vi "MIPI_RFEE_Write and Read Utility.vi"() -> ()   [LabVIEW 2013]
doc: "This VI demonstaits how to write to and read back data from a MIPI device. To run this VI:\n1) Change Resource name to the name of your HSDIO card\n2) The MIPI clock will run at <Sample Clock Rate>/<Oversample Factor>. This is 26 MHz (full rate). If your device should be run at a slower rate, decrease the sample clock rate and (or) increase the oversample rate.\n3. At 104MHz, the RTD value should be ~5 for a 1.5 meter cable. If you are running at a different clock rate or using a different length cable, adjust the RTD Compensation value so the MIPI data is stable at the falling edge of the clock. If you need futher timing adjustment, consider setting the data position to \"Delay from Sample Clock Rising Edge\" and configuring this delay."
uses:
  MIPI_RFFE/Ctrls/Configuration.ctl
  MIPI_RFFE/Ctrls/ClockDataChannels.ctl
  <instrlib>/niHSDIO/niHSDIO.llb/niHSDIO_ctl Sample Clock Source Values (ComboBox).ctl
  <instrlib>/niHSDIO/niHSDIO.llb/niHSDIO_ctl Voltage Logic Family Values (Ring).ctl
  MIPI_RFFE/Ctrls/RegReadWrite.ctl
  <instrlib>/niHSDIO/niHSDIO.llb/niHSDIO_ctl Data Position Values (Ring).ctl
  MIPI_RFFE/Ctrls/ExtendedRegReadWrite.ctl
  <instrlib>/niHSDIO/niHSDIO.llb/niHSDIO Configure Data Voltage Logic Family.vi
  <instrlib>/niHSDIO/niHSDIO.llb/niHSDIO Configure Digital Edge Start Trigger.vi
  <instrlib>/niHSDIO/niHSDIO.llb/niHSDIO Configure Initial State (String).vi
  <instrlib>/niHSDIO/niHSDIO.llb/niHSDIO Configure Idle State (String).vi
  <instrlib>/niHSDIO/niHSDIO.llb/niHSDIO Write Named Waveform (WDT).vi
  <instrlib>/niHSDIO/niHSDIO.llb/niHSDIO Fetch Waveform (WDT).vi
  <vilib>/Waveform/DWDTOps.llb/DWDT Append Digital Signals.vi
panel:
  in  "Filename":string
  in  "Save .HWS?":bool
  in  "file path":path=path "C:/Users/er080167/Documents/AD4125E/Waveforms/Converted Waveforms"
  in  "channel list (all:\"\")":string="4,6"
  in  "delay (0.000)":dbl format="%.3f"
  out "Parity Error":bool
  out "MIPI Data Read from DUT":cluster{"Read Data":u8[]}[](array[cluster])=[{"Read Data"=[128]}] {"Read Data" format="%.0x"}
  in  "Register Read/Write":T1={"Slave Address"=6, "Register"=28, "Data"=128} {"Data" format="%.0x"; "Register" format="%.0x"; "Slave Address" max=15 format="%.0x"}
  in  "RTD Compensation Value":i32=1 min=0 max=29
  out "Digital Waveform Graph":digitalwaveform(graph)={"t0"=timestamp(3585852840.1106524 s since 1904-01-01), "dt"=5e-07, "Y"={"transitions"=[], "data"=[[1, 0, 1, 0], [1, 0, 1, 0], [1, 0, 1, 0], [1, 0, 1, 0], [1, 0, 1, 0], [1, 0, 1, 0], [1, 0, 1, 0], [1, 0, 1, 0], [0, 0, 0, 0], [0, 0, 0, 0], [0, 0, 0, 0], [0, 0, 0, 0], [0, 0, 0, 0], [0, 0, 0, 0], [0, 0, 0, 0], [0, 0, 0, 0], [0, 1, 0, 1], [0, 1, 0, 1], [0, 1, 0, 1], [0, 1, 0, 1], [0, 0, 0, 0], [0, 0, 0, 0], [0, 0, 0, 0], [0, 0, 0, 0], [1, 1, 1, 1], [1, 1, 1, 1], [1, 1, 1, 1], [1, 1, 1, 1], [1, 0, 1, 0], [1, 0, 1, 0], [1, 0, 1, 0], [1, 0, 1, 0], [1, 1, 1, 1], [1, 1, 1, 1], [1, 1, 1, 1], [1, 1, 1, 1], [1, 0, 1, 0], [1, 0, 1, 0], [1, 0, 1, 0], [1, 0, 1, 0], [0, 1, 0, 1], [0, 1, 0, 1], [0, 1, 0, 1], [0, 1, 0, 1], [0, 0, 0, 0], [0, 0, 0, 0], [0, 0, 0, 0], [0, 0, 0, 0], [0, 1, 0, 1], [0, 1, 0, 1], [0, 1, 0, 1], [0, 1, 0, 1], [0, 0, 0, 0], [0, 0, 0, 0], [0, 0, 0, 0], [0, 0, 0, 0], [1, 1, 1, 1], [1, 1, 1, 1], [1, 1, 1, 1], [1, 1, 1, 1], [1, 0, 1, 0], [1, 0, 1, 0], [1, 0, 1, 0], [1, 0, 1, 0], [0, 1, 0, 1], [0, 1, 0, 1], [0, 1, 0, 1], [0, 1, 0, 1], [0, 0, 0, 0], [0, 0, 0, 0], [0, 0, 0, 0], [0, 0, 0, 0], [1, 1, 1, 1], [1, 1, 1, 1], [1, 1, 1, 1], [1, 1, 1, 1], [1, 0, 1, 0], [1, 0, 1, 0], [1, 0, 1, 0], [1, 0, 1, 0], [1, 1, 1, 1], [1, 1, 1, 1], [1, 1, 1, 1], [1, 1, 1, 1], [1, 0, 1, 0], [1, 0, 1, 0], [1, 0, 1, 0], [1, 0, 1, 0], [1, 1, 1, 1], [1, 1, 1, 1], [1, 1, 1, 1], [1, 1, 1, 1], [1, 0, 1, 0], [1, 0, 1, 0], [1, 0, 1, 0], [1, 0, 1, 0], [0, 1, 0, 1], [0, 1, 0, 1], [0, 1, 0, 1], [0, 1, 0, 1], [0, 0, 0, 0], [0, 0, 0, 0], [0, 0, 0, 0], [0, 0, 0, 0], [0, 1, 0, 1], [0, 1, 0, 1], [0, 1, 0, 1], [0, 1, 0, 1], [0, 0, 0, 0], [0, 0, 0, 0], [0, 0, 0, 0], [0, 0, 0, 0], [1, 1, 1, 1], [1, 1, 1, 1], [1, 1, 1, 1], [1, 1, 1, 1], [1, 0, 1, 0], [1, 0, 1, 0], [1, 0, 1, 0], [1, 0, 1, 0], [1, 1, 1, 1], [1, 1, 1, 1], [1, 1, 1, 1], [1, 1, 1, 1], [1, 0, 1, 0], [1, 0, 1, 0], [1, 0, 1, 0], [1, 0, 1, 0], [0, 1, 0, 1], [0, 1, 0, 1], [0, 1, 0, 1], [0, 1, 0, 1], [0, 0, 0, 0], [0, 0, 0, 0], [0, 0, 0, 0], [0, 0, 0, 0], [0, 1, 0, 1], [0, 1, 0, 1], [0, 1, 0, 1], [0, 1, 0, 1], [0, 0, 0, 0], [0, 0, 0, 0], [0, 0, 0, 0], [0, 0, 0, 0], [0, 1, 0, 1], [0, 1, 0, 1], [0, 1, 0, 1], [0, 1, 0, 1], [0, 0, 0, 0], [0, 0, 0, 0], [0, 0, 0, 0], [0, 0, 0, 0], [0, 1, 0, 1], [0, 1, 0, 1], [0, 1, 0, 1], [0, 1, 0, 1], [0, 0, 0, 0], [0, 0, 0, 0], [0, 0, 0, 0], [0, 0, 0, 0], [0, 1, 0, 1], [0, 1, 0, 1], [0, 1, 0, 1], [0, 1, 0, 1], [0, 0, 0, 0], [0, 0, 0, 0], [0, 0, 0, 0], [0, 0, 0, 0], [0, 1, 0, 1], [0, 1, 0, 1], [0, 1, 0, 1], [0, 1, 0, 1], [0, 0, 0, 0], [0, 0, 0, 0], [0, 0, 0, 0], [0, 0, 0, 0], [0, 1, 0, 1], [0, 1, 0, 1], [0, 1, 0, 1], [0, 1, 0, 1], [0, 0, 0, 0], [0, 0, 0, 0], [0, 0, 0, 0], [0, 0, 0, 0], [0, 1, 0, 1], [0, 1, 0, 1], [0, 1, 0, 1], [0, 1, 0, 1], [0, 0, 0, 0], [0, 0, 0, 0], [0, 0, 0, 0], [0, 0, 0, 0], [0, 1, 0, 1], [0, 1, 0, 1], [0, 1, 0, 1], [0, 1, 0, 1], [0, 0, 0, 0], [0, 0, 0, 0], [0, 0, 0, 0], [0, 0, 0, 0], [1, 0, 1, 0], [1, 0, 1, 0], [1, 0, 1, 0], [1, 0, 1, 0], [1, 0, 1, 0], [1, 0, 1, 0], [1, 0, 1, 0], [1, 0, 1, 0], [0, 0, 0, 0], [0, 0, 0, 0], [0, 0, 0, 0], [0, 0, 0, 0], [0, 0, 0, 0], [0, 0, 0, 0], [0, 0, 0, 0], [0, 0, 0, 0], [0, 1, 0, 1], [0, 1, 0, 1], [0, 1, 0, 1], [0, 1, 0, 1], [0, 0, 0, 0], [0, 0, 0, 0], [0, 0, 0, 0], [0, 0, 0, 0], [1, 1, 1, 1], [1, 1, 1, 1], [1, 1, 1, 1], [1, 1, 1, 1], [1, 0, 1, 0], [1, 0, 1, 0], [1, 0, 1, 0], [1, 0, 1, 0], [1, 1, 1, 1], [1, 1, 1, 1], [1, 1, 1, 1], [1, 1, 1, 1], [1, 0, 1, 0], [1, 0, 1, 0], [1, 0, 1, 0], [1, 0, 1, 0], [0, 1, 0, 1], [0, 1, 0, 1], [0, 1, 0, 1], [0, 1, 0, 1], [0, 0, 0, 0], [0, 0, 0, 0], [0, 0, 0, 0], [0, 0, 0, 0], [0, 1, 0, 1], [0, 1, 0, 1], [0, 1, 0, 1], [0, 1, 0, 1], [0, 0, 0, 0], [0, 0, 0, 0], [0, 0, 0, 0], [0, 0, 0, 0], [1, 1, 1, 1], [1, 1, 1, 1], [1, 1, 1, 1], [1, 1, 1, 1], [1, 0, 1, 0], [1, 0, 1, 0], [1, 0, 1, 0], [1, 0, 1, 0], [1, 1, 1, 1], [1, 1, 1, 1], [1, 1, 1, 1], [1, 1, 1, 1], [1, 0, 1, 0], [1, 0, 1, 0], [1, 0, 1, 0], [1, 0, 1, 0], [1, 1, 1, 1], [1, 1, 1, 1], [1, 1, 1, 1], [1, 1, 1, 1], [1, 0, 1, 0], [1, 0, 1, 0], [1, 0, 1, 0], [1, 0, 1, 0], [1, 1, 1, 1], [1, 1, 1, 1], [1, 1, 1, 1], [1, 1, 1, 1], [1, 0, 1, 0], [1, 0, 1, 0], [1, 0, 1, 0], [1, 0, 1, 0], [1, 1, 1, 1], [1, 1, 1, 1], [1, 1, 1, 1], [1, 1, 1, 1], [1, 0, 1, 0], [1, 0, 1, 0], [1, 0, 1, 0], [1, 0, 1, 0], [0, 1, 0, 1], [0, 1, 0, 1], [0, 1, 0, 1], [0, 1, 0, 1], [0, 0, 0, 0], [0, 0, 0, 0], [0, 0, 0, 0], [0, 0, 0, 0], [0, 1, 0, 1], [0, 1, 0, 1], [0, 1, 0, 1], [0, 1, 0, 1], [0, 0, 0, 0], [0, 0, 0, 0], [0, 0, 0, 0], [0, 0, 0, 0], [0, 1, 0, 1], [0, 1, 0, 1], [0, 1, 0, 1], [0, 1, 0, 1], [0, 0, 0, 0], [0, 0, 0, 0], [0, 0, 0, 0], [0, 0, 0, 0], [0, 1, 0, 1], [0, 1, 0, 1], [0, 1, 0, 1], [0, 1, 0, 1], [0, 0, 0, 0], [0, 0, 0, 0], [0, 0, 0, 0], [0, 0, 0, 0], [1, 1, 5, 1], [1, 1, 5, 1], [1, 1, 5, 1], [1, 1, 5, 1], [1, 0, 4, 0], [1, 0, 5, 0], [1, 0, 5, 0], [1, 0, 5, 0], [0, 1, 5, 1], [0, 1, 5, 1], [0, 1, 5, 1], [0, 1, 5, 1], [0, 0, 3, 0], [0, 0, 5, 0], [0, 0, 5, 0], [0, 0, 5, 0], [0, 1, 5, 1], [0, 1, 5, 1], [0, 1, 5, 1], [0, 1, 5, 1], [0, 0, 3, 0], [0, 0, 5, 0], [0, 0, 5, 0], [0, 0, 5, 0], [0, 1, 5, 1], [0, 1, 5, 1], [0, 1, 5, 1], [0, 1, 5, 1], [0, 0, 3, 0], [0, 0, 5, 0], [0, 0, 5, 0], [0, 0, 5, 0], [0, 1, 5, 1], [0, 1, 5, 1], [0, 1, 5, 1], [0, 1, 5, 1], [0, 0, 3, 0], [0, 0, 5, 0], [0, 0, 5, 0], [0, 0, 5, 0], [0, 1, 5, 1], [0, 1, 5, 1], [0, 1, 5, 1], [0, 1, 5, 1], [0, 0, 3, 0], [0, 0, 5, 0], [0, 0, 5, 0], [0, 0, 5, 0], [0, 1, 5, 1], [0, 1, 5, 1], [0, 1, 5, 1], [0, 1, 5, 1], [0, 0, 3, 0], [0, 0, 5, 0], [0, 0, 5, 0], [0, 0, 5, 0], [0, 1, 5, 1], [0, 1, 5, 1], [0, 1, 5, 1], [0, 1, 5, 1], [0, 0, 3, 0], [0, 0, 5, 0], [0, 0, 5, 0], [0, 0, 5, 0], [0, 1, 5, 1], [0, 1, 5, 1], [0, 1, 5, 1], [0, 1, 5, 1], [0, 0, 3, 0], [0, 0, 5, 0], [0, 0, 5, 0], [0, 0, 5, 0], [0, 1, 0, 1], [0, 1, 0, 1], [0, 1, 0, 1], [0, 1, 0, 1], [0, 0, 0, 0], [0, 0, 0, 0], [0, 0, 0, 0], [0, 0, 0, 0]]}}
  in  "Configuratation":T2={"Samples to Allocate"=10000, "Oversample Factor"=1, "Clock Channel"=enum."0", "Data Channel"=enum."1"} {"Oversample Factor" min=1 max=254; "Samples to Allocate" min=1}
  out "Number of Sample Errors Read":i32
  in  "Sample Clock Rate":dbl=2000000.0 format="%#_6p"
  in  "Resource name":refnum<k15>="6556_0"
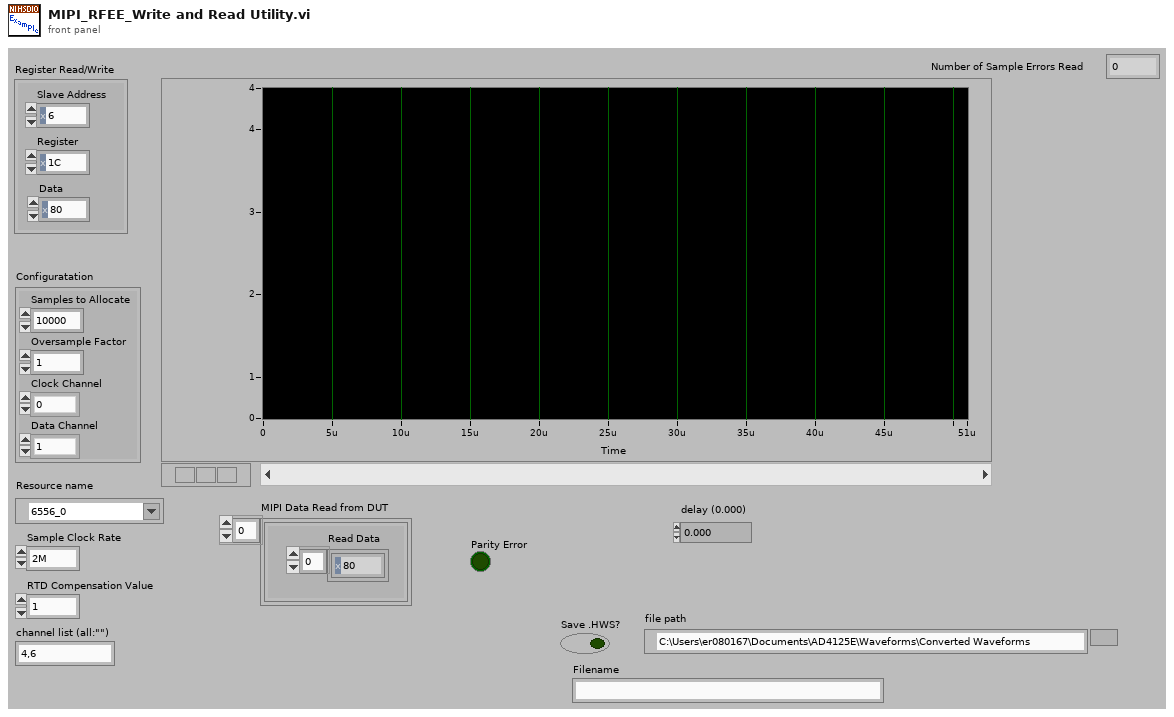
[diagram p1: front panel]
types:
  T1 = cluster{"Slave Address":u8, "Register":u8, "Data":u8}
  T2 = typedef "Configuration.ctl" = cluster{"Samples to Allocate":i32, "Oversample Factor":u8, "Clock Channel":T3, "Data Channel":T3}
  T3 = typedef "ClockDataChannels.ctl" = enum16{"0", "1"}
  T4 = typedef "niHSDIO_ctl Data Position Values (Ring).ctl" = i32
  T5 = typedef "RegReadWrite.ctl" = cluster{"Slave Address":u8, "Register":u8, "Data":u8}
  T6 = typedef "niHSDIO_ctl Voltage Logic Family Values (Ring).ctl" = i32
  T7 = typedef "niHSDIO_ctl Sample Clock Source Values (ComboBox).ctl" = string
  T8 = typedef "RFFE_Data.ctl" = cluster{"Clock Channel":T3, "Data Channel":T3, "Oversample Factor":u8, "Zero Array":u8[], "One Array":u8[], "Z Array ":u8[], "H Array":u8[], "L Array":u8[], "X Array":u8[], "Toggle (high to low)":u8[]}
  T9 = typedef "ExtendedRegReadWrite.ctl" = cluster{"Slave Address":u8, "Register":u8, "Data":u8[]}
  T10 = typedef "ReadInfo.ctl" = cluster{"Expected Value(s)":u8[], "Compare Locations":u32[]}
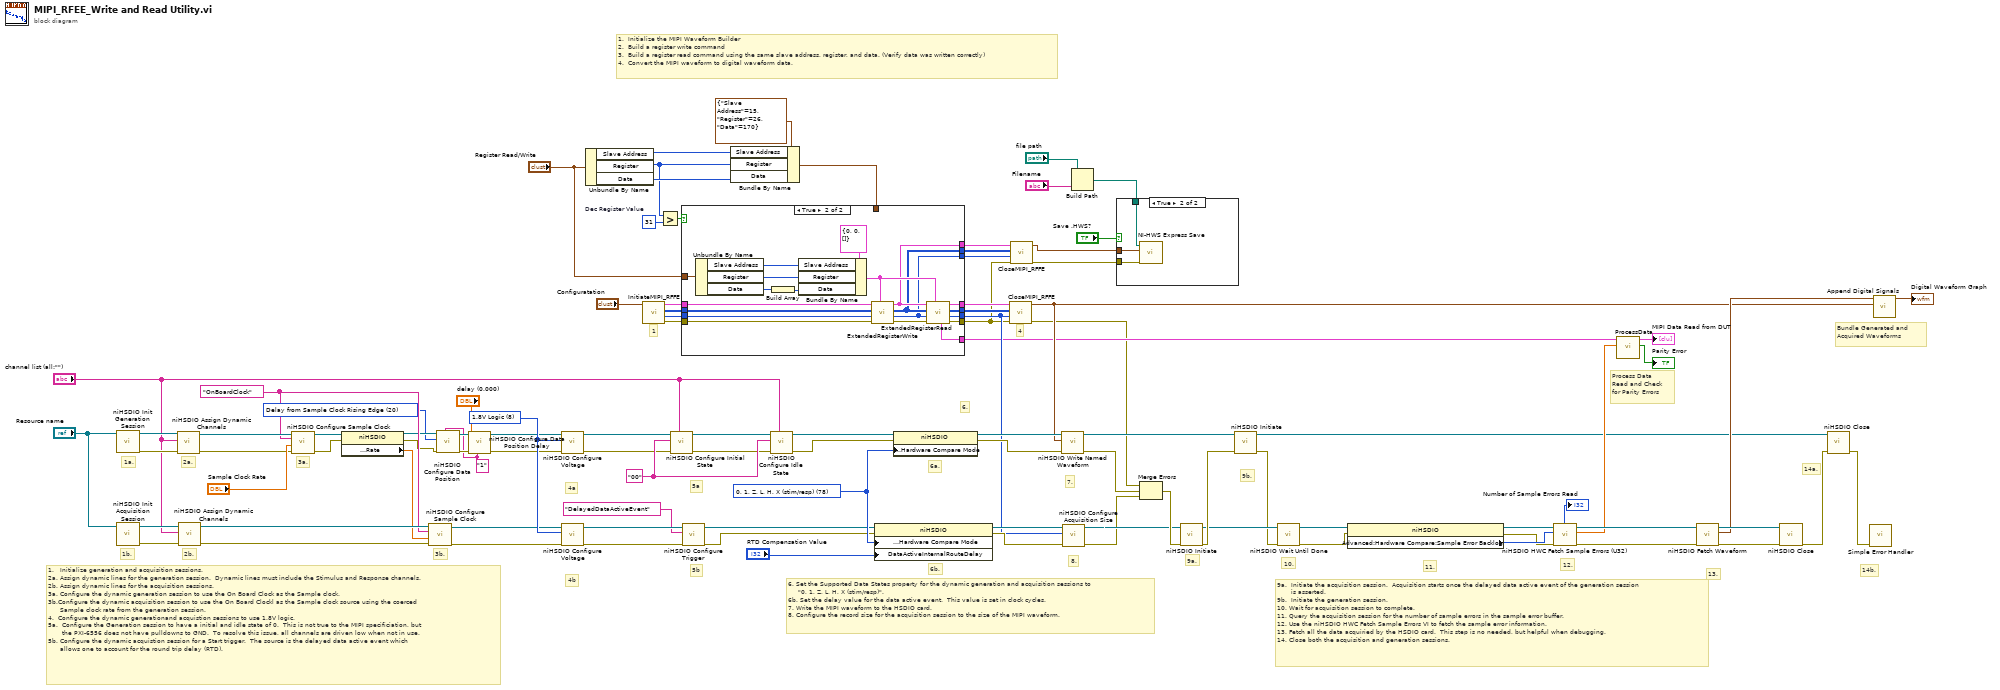
[diagram p0: block diagram]
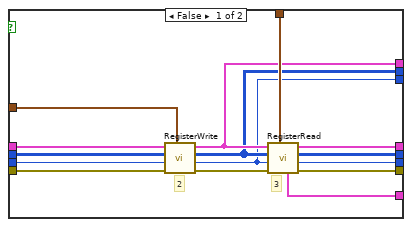
[diagram p3: hidden frame]
diagram:
  w16 = u8 31  # Dec Register Value
  w22 = T4 20 items=["Sample Clock Rising Edge"=18, "Sample Clock Falling Edge"=19, "Delay from Sample Clock Rising Edge"=20] ("position (rising edge)")
  w21 = "1" ("channel list (all:\"\")")
  w37 = "00" ("idle state")
  w68 = T6 8 items=["5.0V Logic"=5, "3.3V Logic"=6, "2.5V Logic"=7, "1.8V Logic"=8, "1.5V Logic"=80, "1.2V Logic"=81] ("logic family (3.3V logic)")
  w85 = 78 items=["0, 1 (binary)"=77, "0, 1, Z (tristate)"=83, "0, 1, Z, L, H, X (stim/resp)"=78, "L, H, X (resp only)"=79] ("Advanced:Supported Data States")
  w53 = T7 "OnBoardClock" ("clock source (on board clock)")
  # "4"
  # "1"
  # "1.  Initialize the MIPI Waveform Builder\n2.  Build a register write command\n3.  Build a register read command using the same slave address, register, and data. (Verify data was written correctly)\n4.  Convert the MIPI waveform to digital waveform data."
  # "Bundle Generated and Acquired Waveforms"
  # "5a"
  # "Process Data Read and Check for Parity Errors"
  # "4b"
  # "4a"
  # "13."
  # "6. Set the Supported Data States property for the dynamic generation and acquisition sessions to \n     \"0, 1, Z, L, H, X (stim/resp)\".\n6b. Set the delay value for the data active event.  This value is set in clock cycles.\n7. Write the MIPI waveform to the HSDIO card.\n8. Configure the record size for the acquisition session to the size of the MIPI waveform."
  # "6."
  # "1.   Initialize generation and acquisition sessions.\n2a. Assign dynamic lines for the generation session.  Dynamic lines must include the Stimulus and Response channels.\n2b. Assign dynamic lines for the acquisition sessions.\n3a. Configure the dynamic generation session to use the On Board Clock as the Sample clock.\n3b.Configure the dynamic acquisition session to use the On Board Clockl as the Sample clock source using the coerced \n      Sample clock rate from the generation session.\n4.  Configure the dynamic generationand acquistion sessions to use 1.8V logic.\n5a.  Configure the Generation session to have a initial and idle state of 0.  This is not true to the MIPI specificiation, but\n       the PXI-6556 does not have pulldowns to GND.  To resolve this issue, all channels are driven low when not in use.\n5b. Configure the dynamic acquistion session for a Start trigger.  The source is the delayed data active event which\n      allows one to account for the round trip delay (RTD)."
  # "14b."
  # "12."
  # "11."
  # "10."
  # "9b."
  # "9a."
  # "9a.  Initiate the acquisition session.  Acquisition starts once the delayed data active event of the generation session\n       is asserted. \n9b.  Initiate the generation session.\n10. Wait for acquisition session to complete.\n11. Query the acquisition session for the number of sample errors in the sample error buffer.\n12. Use the niHSDIO HWC Fetch Sample Errors VI to fetch the sample error information.\n13. Fetch all the data acquiried by the HSDIO card.  This step is no needed, but helpful when debugging.\n14. Close both the acquisition and generation sessions."
  # "8."
  # "7."
  # "6b."
  # "6a."
  # "5b"
  # "3b."
  # "3a."
  # "2b."
  # "2a."
  # "1b."
  # "1a."
  # "14a."
  n1 = call <instrlib>:"niHSDIO Init Generation Session.vi"("resource name"="Resource name") -> ("error out"=w56:errorcluster, "instrument handle out"=w57:refnum<k15>)  [unwired: 9 in]
  n2 = call <instrlib>:"niHSDIO Init Acquisition Session.vi"("resource name"="Resource name") -> ("error out"=w60:errorcluster, "instrument handle out"=w96:refnum<k15>)  [unwired: 9 in]
  n3 = call <instrlib>:"niHSDIO Assign Dynamic Channels.vi"("error in (no error)"=w56, "channel list (all:\"\")"="channel list (all:\"\")", "instrument handle"=w57) -> ("error out"=w83:errorcluster, "instrument handle out"=w84:refnum<k15>)  [unwired: 7 in]
  n4 = call <instrlib>:"niHSDIO Assign Dynamic Channels.vi"("error in (no error)"=w60, "channel list (all:\"\")"="channel list (all:\"\")", "instrument handle"=w96) -> ("error out"=w75:errorcluster, "instrument handle out"=w76:refnum<k15>)  [unwired: 7 in]
  n5 = call <instrlib>:"niHSDIO Configure Sample Clock.vi"("error in (no error)"=w83, "clock rate (50MHz)"="Sample Clock Rate", "clock source (on board clock)"=w53, "instrument handle"=w84) -> ("error out"=w54:errorcluster, "instrument handle out"=w55:refnum<k15>)  [unwired: 6 in]
  n6 = property on="Property Node" class="niHSDIO"(reference=w55, error in=w54) -> (reference out=w24:refnum<k15>, error out=w23:errorcluster, "Timing:Sample Clock:Rate"=w72:dbl)
  n7 = call <instrlib>:"niHSDIO Configure Sample Clock.vi"("error in (no error)"=w75, "clock rate (50MHz)"=w72, "clock source (on board clock)"=w53, "instrument handle"=w76) -> ("error out"=w52:errorcluster, "instrument handle out"=w51:refnum<k15>)  [unwired: 6 in]
  n8 = call <instrlib>:"niHSDIO Configure Data Position.vi"("channel list (all:\"\")"=w21, "error in (no error)"=w23, "position (rising edge)"=w22, "instrument handle"=w24) -> ("error out"=w26:errorcluster, "instrument handle out"=w25:refnum<k15>)  [unwired: 6 in]
  n9 = call <instrlib>:"niHSDIO Configure Data Position Delay.vi"("channel list (all:\"\")"=w21, "error in (no error)"=w26, "delay (0.000)"="delay (0.000)", "instrument handle"=w25) -> ("error out"=w29:errorcluster, "instrument handle out"=w28:refnum<k15>)  [unwired: 6 in]
  n10 = call-poly <instrlib>:"niHSDIO Configure Voltage.vi"("error in (no error)"=w29, "logic family (3.3V logic)"=w68, "instrument handle"=w28) -> ("error out"=w33:errorcluster, "instrument handle out"=w34:refnum<k15>)  [unwired: 7 in]
  n11 = call-poly <instrlib>:"niHSDIO Configure Voltage.vi"("error in (no error)"=w52, "logic family (3.3V logic)"=w68, "instrument handle"=w51) -> ("error out"=w49:errorcluster, "instrument handle out"=w50:refnum<k15>)  [unwired: 7 in]
  n12 = Unbundle By Name("Register Read/Write") -> ("Slave Address"=w19:u8, "Register"=w1:u8, "Data"=w15:u8)
  n13 = call "InitiateMIPI_RFFE.vi"("Configuratation In"="Configuratation") -> ("error out"=w67:errorcluster, "Number of Samples Out"=w66:i32, "Data Array"=w65:u8[][], "RFFE_Data"=w63:T8)  [unwired: 7 in]
  n14 = Greater?(x=w1, y=w16) -> (0:w14:bool)
  n15 = call-poly <instrlib>:"niHSDIO Configure Initial State.vi"("channel list"="channel list (all:\"\")", "error in (no error)"=w33, "initial state"=w37, "instrument handle"=w34) -> ("error out"=w36:errorcluster, "instrument handle out"=w35:refnum<k15>)  [unwired: 6 in]
  n16 = call-poly <instrlib>:"niHSDIO Configure Trigger.vi"("error in (no error)"=w49, "source (PFI 0)"="DelayedDataActiveEvent" ("channel list (all:\"\")"), "instrument handle"=w50) -> ("error out"=w45:errorcluster, "instrument handle out"=w48:refnum<k15>)  [unwired: 7 in]
  n17 = Bundle By Name(cluster=T5 {"Slave Address"=15, "Register"=26, "Data"=170} ("Register Read/Write"), "Slave Address"=w19, "Register"=w1, "Data"=w15) -> (w18:T5)
  n18 = case shown="True" w14 {
    tunnel: w67 -> [w115 w135]
    tunnel: w66 -> [w114 w132]
    tunnel: w65 -> [w113 w133]
    tunnel: w63 -> [w112 w134]
    tunnel: [w110 w121] -> w43
    tunnel: [w109 w122] -> w42
    tunnel: [w108 w123] -> w41
    tunnel: [w107 w124] -> w9
    tunnel: [w106 w119] -> w40
    tunnel: w18 -> [w105 _]
    tunnel: "Register Read/Write" -> [w104 w130]
    tunnel: [w103 w118] -> w12
    tunnel: [w102 w117] -> w11
    tunnel: [w101 w116] -> w10
    frame False {
      # "3"
      # "2"
      n19 = call "RegisterWrite.vi"("Write Data"=w104, "error in (no error)"=w115, "Number of Samples In"=w114, "Data Array"=w113, "RFFE_Data"=w112) -> ("error out"=w111:errorcluster, "Number of Samples Out"=w101:i32, "Data Array Out"=w102:u8[][], "Configuratation Out"=w103:T8)  [unwired: 3 in]
      n20 = call "RegisterRead.vi"("Register Read/Write"=w105, "error in (no error)"=w111, "Number of Samples In"=w101, "Data Array"=w102, "RFFE_Data In"=w103) -> ("error out"=w107:errorcluster, "Number of Samples Out out"=w108:i32, "Data Array Out"=w109:u8[][], "RFFE_Data Out"=w110:T8, "Compare Bits Out"=w106:T10[])  [unwired: 2 in]
    }
    frame True {
      n21 = Unbundle By Name(w130) -> ("Slave Address"=w129:u8, "Register"=w128:u8, "Data"=w127:u8)
      n22 = Build Array(w127) -> (w126:u8[])
      n23 = Bundle By Name(cluster=T9 {"Slave Address"=0, "Register"=0, "Data"=[]} ("Extended Read/Write"), "Slave Address"=w129, "Register"=w128, "Data"=w126) -> (w120:T9)
      n24 = call "ExtendedRegisterWrite.vi"("Extended Read/Write"=w120, "error in (no error)"=w135, "Number of Samples In"=w132, "Data Array"=w133, "RFFE_Data In"=w134) -> ("error out"=w125:errorcluster, "Number of Samples Out"=w116:i32, "Data Array Out"=w117:u8[][], "RFFE_Data Out"=w118:T8)  [unwired: 3 in]
      n25 = call "ExtendedRegisterRead.vi"("Extended Read/Write"=w120, "error in (no error)"=w125, "Number of Samples In"=w116, "Data Array"=w117, "RFFE_Data In"=w118) -> ("error out"=w124:errorcluster, "Number of Samples Out out"=w123:i32, "Data Array Out"=w122:u8[][], "RFFE_Data Out"=w121:T8, "Compare Bits Out"=w119:T10[])  [unwired: 2 in]
    }
  }
  n26 = call-poly <instrlib>:"niHSDIO Configure Idle State.vi"("channel list"="channel list (all:\"\")", "error in (no error)"=w36, "idle state"=w37, "instrument handle"=w35) -> ("error out"=w32:errorcluster, "instrument handle out"=w31:refnum<k15>)  [unwired: 6 in]
  n27 = property on="Property Node" class="niHSDIO"(reference=w48, error in=w45, "Advanced:Hardware Compare:Hardware Compare Mode"=w85, "DataActiveInternalRouteDelay"="RTD Compensation Value") -> (reference out=w80:refnum<k15>, error out=w79:errorcluster)
  n28 = property on="Property Node" class="niHSDIO"(reference=w31, error in=w32, "Advanced:Hardware Compare:Hardware Compare Mode"=w85) -> (reference out=w82:refnum<k15>, error out=w81:errorcluster)
  n29 = call "CloseMIPI_RFFE.vi"("error in (no error)"=w9, "Number of Samples"=w41, "Data Array"=w42, "RFFE_Data"=w43) -> ("error out"=w13:errorcluster, "Digital Waveform"=w44:digitalwaveform)  [unwired: 6 in]
  n30 = call "CloseMIPI_RFFE.vi"("error in (no error)"=w9, "Number of Samples"=w10, "Data Array"=w11, "RFFE_Data"=w12) -> ("error out"=w6:errorcluster, "Digital Waveform"=w7:digitalwaveform)  [unwired: 6 in]
  n31 = call-poly <instrlib>:"niHSDIO Write Named Waveform.vi"("error in (no error)"=w81, "data"=w44, "instrument handle"=w82) -> ("error out"=w73:errorcluster, "instrument handle out"=w87:refnum<k15>)  [unwired: 7 in]
  n32 = call <instrlib>:"niHSDIO Configure Acquisition Size.vi"("error in (no error)"=w79, "samples per record (1000 samples)"=w41, "instrument handle"=w80) -> ("error out"=w74:errorcluster, "instrument handle out"=w78:refnum<k15>)  [unwired: 7 in]
  n33 = Build Path(base path="file path", name or relative path="Filename") -> (appended path=w2:path)
  n34 = case shown="True" "Save .HWS?" {
    tunnel: w7 -> [_ w138]
    tunnel: w6 -> [_ w137]
    tunnel: w2 -> [_ w136]
    frame False {
    }
    frame True {
      n35 = call "NI-HWS Express Save"("error in"=w137, "digital waveform"=w138, "file path"=w136) -> ()  [unwired: 8 in, 1 out]
    }
  }
  n36 = Merge Errors(w13, w73, w74) -> (w86:errorcluster)
  n37 = call <instrlib>:"niHSDIO Initiate.vi"("error in (no error)"=w86, "instrument handle"=w78) -> ("error out"=w95:errorcluster, "instrument handle out"=w93:refnum<k15>)  [unwired: 8 in]
  n38 = call <instrlib>:"niHSDIO Initiate.vi"("error in (no error)"=w95, "instrument handle"=w87) -> ("error out"=w91:errorcluster, "instrument handle out"=w58:refnum<k15>)  [unwired: 8 in]
  n39 = call <instrlib>:"niHSDIO Wait Until Done.vi"("error in (no error)"=w91, "instrument handle"=w93) -> ("error out"=w90:errorcluster, "instrument handle out"=w92:refnum<k15>)  [unwired: 8 in]
  n40 = property on="Property Node" class="niHSDIO"(reference=w92, error in=w90) -> (reference out=w89:refnum<k15>, error out=w88:errorcluster, "Advanced:Hardware Compare:Sample Error Backlog"=w97:i32)
  n41 = call <instrlib>:"niHSDIO HWC Fetch Sample Errors (U32).vi"("error in (no error)"=w88, "sample errors  to read"=w97, "instrument handle"=w89) -> ("error out"=w71:errorcluster, "sample numbers"=w61:dbl[], "instrument handle out"=w70:refnum<k15>, "number of sample errors read"=→"Number of Sample Errors Read":i32)  [unwired: 3 in, 2 out]
  n42 = call "ProcessData.vi"("Error Loacations"=w61, "Read Info"=w40) -> ("Parity Error"=→"Parity Error":bool, "Read MIPI Data"=→"MIPI Data Read from DUT":cluster{"Read Data":u8[]}[])  [unwired: 8 in]
  n43 = call-poly <instrlib>:"niHSDIO Fetch Waveform.vi"("error in (no error)"=w71, "instrument handle"=w70) -> ("error out"=w59:errorcluster, "data"=w64:digitalwaveform, "instrument handle out"=w99:refnum<k15>)  [unwired: 6 in, 1 out]
  n44 = call <instrlib>:"niHSDIO Close.vi"("error in (no error)"=w59, "instrument handle"=w99) -> ("error out"=w100:errorcluster)  [unwired: 9 in]
  n45 = call <instrlib>:"niHSDIO Close.vi"("error in (no error)"=w100, "instrument handle"=w58) -> ("error out"=w8:errorcluster)  [unwired: 9 in]
  n46 = call <vilib>:"Simple Error Handler.vi"("error in (no error)"=w8) -> ()  [unwired: 4 in, 5 out]
  n47 = call-poly <vilib>:"Append Digital Signals.vi"("digital waveform (low bits)"=w44, "digital waveform (high bits)"=w64) -> ("digital waveform out"=→"Digital Waveform Graph":digitalwaveform)  [unwired: 8 in, 1 out]
